vi "Main.vi"() -> ()   [LabVIEW 2025]
uses:
  10416e7f-0477-4853-a6bb-a8675e9e76fc.vi
panel:
  out "River":u16[][](array[ring]) caption="Tiles"
  out "RiverIndex":u16
  out "MountainIndex":u16
  out "String":string
  out "Mountain":u16[](array[numeric])
  out "Ring":u16(ring)
  in  "Buttons":bool[](array[boolean])
  out "Hand":u16[](array[ring])
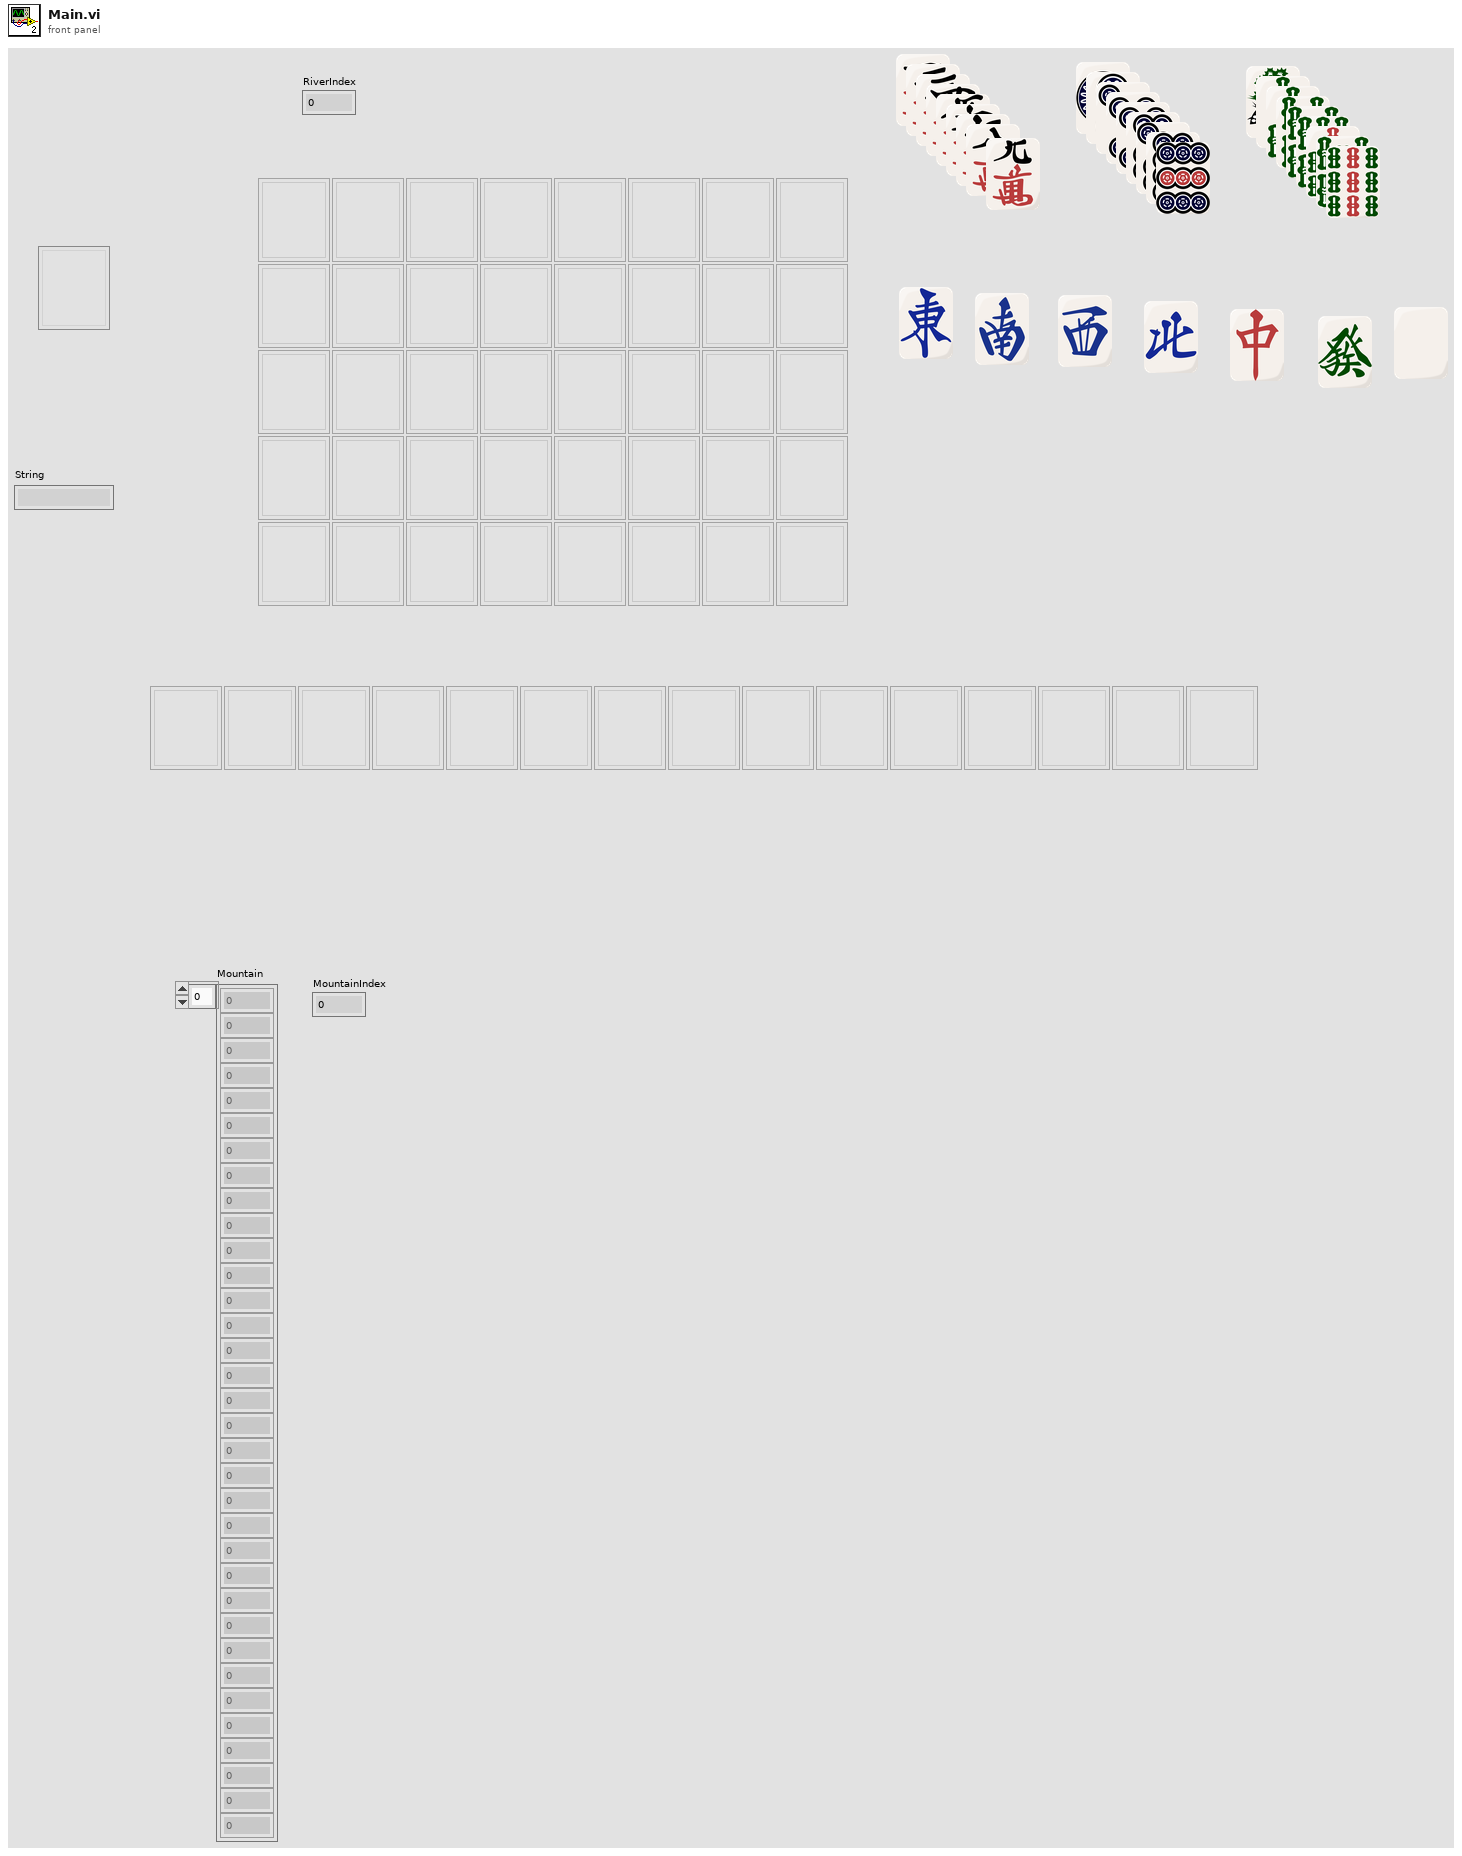
[diagram p1: front panel]
types:
  T1 = typedef "LVPositionTypeDef.ctl" = cluster{"Left":i32, "Top":i32}
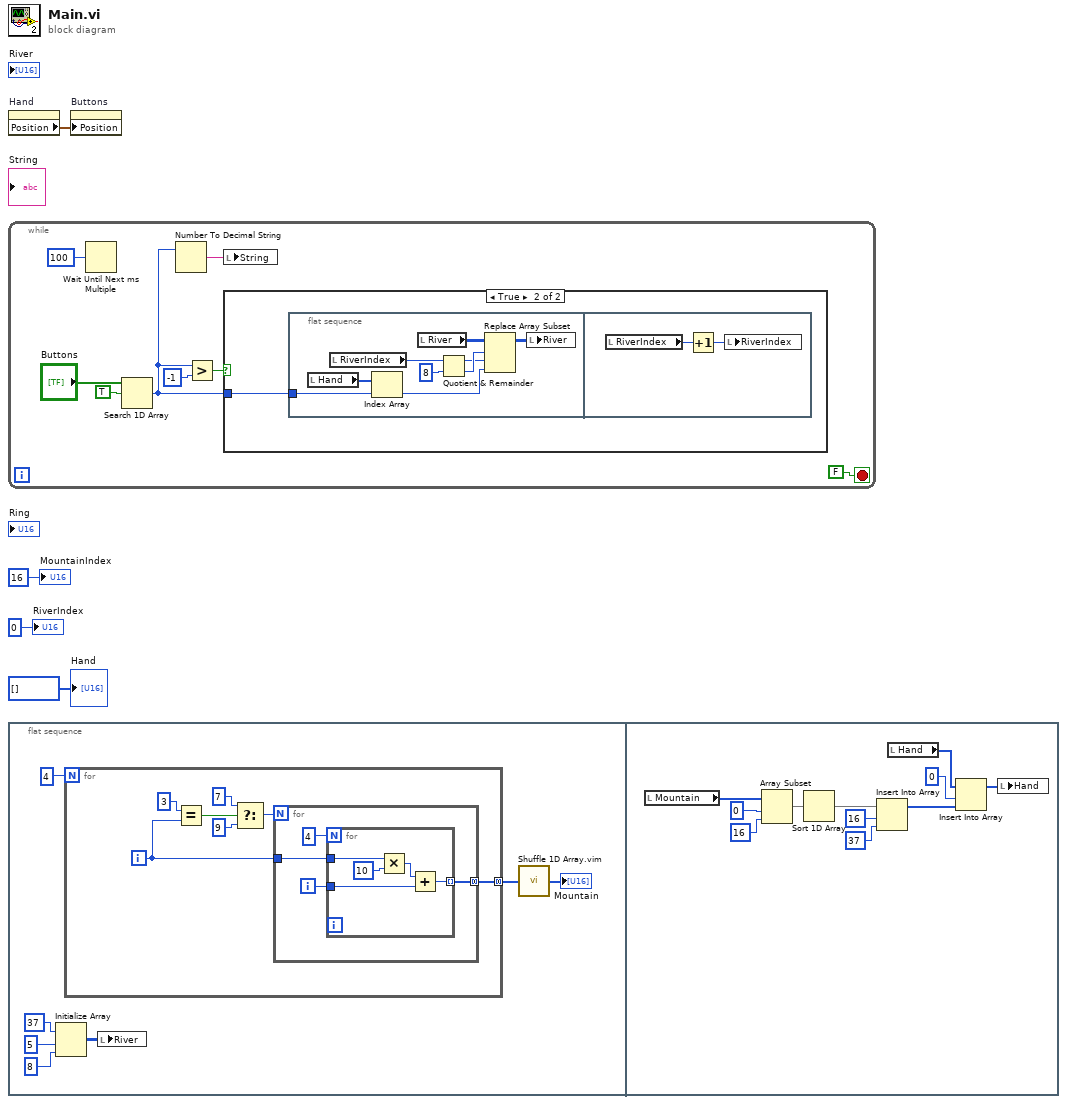
[diagram p0: block diagram]
diagram:
  n1 = property on="Hand" class="Arr (strict)"() -> ("Position"=w1:T1)  [unwired: 2 in, 2 out]
  n2 = while {
    stop <- FALSE stop-if-true
    n3 = Wait Until Next ms Multiple(millisecond multiple=100) -> ()  [unwired: 1 out]
    n4 = Search 1D Array(1D array="Buttons", element=TRUE) -> (index of element=w6:i32)  [unwired: 1 in]
    n5 = Number To Decimal String(number=w6) -> (decimal integer string=w5:string)  [unwired: 1 in]
    n6 = Greater?(x=w6, y=-1) -> (0:w8:bool)
    n7 = local write "String"(w5) -> ()
    n8 = case shown="True" w8 {
      tunnel: w6 -> [_ w13]
      frame False {
      }
      frame True {
        n9 = flat-sequence {
          tunnel: w13 -> [w19]
          frame #0 {
            n10 = local read "Hand"() -> (w18:u16[])
            n11 = local read "RiverIndex"() -> (w17:u16)
            n12 = Index Array(array=w18, index=w19) -> (element=w20:u16)
            n13 = local read "River"() -> (w21:u16[][])
            n14 = Quotient & Remainder(x=w17, y=8) -> (x-y*floor(x/y)=w15:i32, floor(x/y)=w16:i32)
            n15 = Replace Array Subset(array=w21, new element=w20, index (row)=w16, index (col)=w15) -> (w22:u16[][])
            n16 = local write "River"(w22) -> ()
          }
          frame #1 {
            n17 = local read "RiverIndex"() -> (w23:u16)
            n18 = Increment(x=w23) -> (x+1=w24:u16)
            n19 = local write "RiverIndex"(w24) -> ()
          }
        }
      }
    }
  }
  n20 = flat-sequence {
    frame #0 {
      n21 = Initialize Array(37, 5, 8) -> (w25:i32[][])
      n22 = for {
        N: 4 -> [_]
        tunnel: [w35] -> w30 mode=concatenating
        i -> [w33]
        n23 = Equal?(x=3, y=w33) -> (x = y?=w34:bool)
        n24 = Select(t=7, s=w34, f=9) -> (s? t:f=w37:i32)
        n25 = for {
          N: w37 -> [_]
          tunnel: w33 -> [w42]
          tunnel: [w40] -> w35 mode=concatenating
          i -> [w41]
          n26 = for {
            N: 4 -> [_]
            tunnel: w42 -> [w45]
            tunnel: w41 -> [w44]
            tunnel: [w43] -> w40 mode=indexing
            n27 = Multiply(x=w45, y=10) -> (x*y=w47:i32)
            n28 = Add(x=w47, y=w44) -> (x+y=w43:i32)
          }
        }
      }
      n29 = local write "River"(w25) -> ()
      n30 = call "Shuffle 1D Array.vim"("array"=w30) -> ("shuffled array"=→"Mountain":i32[])  [unwired: 4 in]
    }
    frame #1 {
      n31 = local read "Mountain"() -> (w57:u16[])
      n32 = Array Subset(array=w57, index=0, length=16) -> (w49:u16[])
      n33 = Sort 1D Array(array=w49) -> (sorted array=w48:u16[])
      n34 = Insert Into Array(array=w48, index=16, new element=37) -> (w54:u16[])
      n35 = local read "Hand"() -> (w58:u16[])
      n36 = Insert Into Array(array=w58, index=0, new element=w54) -> (w50:u16[])
      n37 = local write "Hand"(w50) -> ()
    }
  }
  n38 = property on="Buttons" class="Arr (strict)"("Position"=w1) -> ()  [unwired: 2 in, 2 out]
  "MountainIndex" <- 16
  "RiverIndex" <- 0
  "Hand" <- i32[] []
